vi "MultU8.vi"(4 "y":u8, 5 "x":u8) -> (1 "x*y":u8, 2 "Overflow?":bool)   [LabVIEW 2017, in "GPOverflow.lvlib"]
doc: "Multiplies <B>x</B> with <B>y</B> keeping track of numeric overflow.\n\n<B>Overflow?</B> will be True if positive or negative overflow occurred. The output will saturate in case of overflow.\n\nThis VI is inlined.\n\nSteen Schmidt\nGPower\n8/8 2013"
uses:
  GPOverflow.lvlib
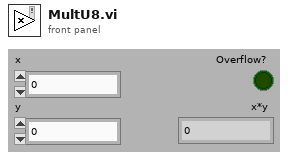
[diagram p1: front panel]
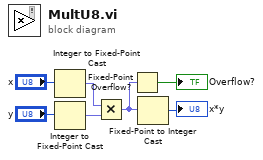
[diagram p0: block diagram]
diagram:
  n1 = Integer to Fixed-Point Cast(integer="x") -> (fixed-point=w5:fxp<+,8,8>)  [unwired: 1 in]
  n2 = Integer to Fixed-Point Cast(integer="y") -> (fixed-point=w4:fxp<+,8,8>)  [unwired: 1 in]
  n3 = Multiply(x=w5, y=w4) -> (x*y=w3:fxp<+,8,8>)
  n4 = Fixed-Point Overflow?(1:w3) -> (0:→"Overflow?":bool)
  n5 = Fixed-Point to Integer Cast(1:w3) -> (0:→"x*y":u8)
